vi "bats.parser.test.AddOrderLong.add.oneOrder.vi"(10 "Expected OrderBook.Command[]":T2[](array[typedef])=[{"type"=enum."AddOrder", "side"=66, "orderId "=2319688266934735439, "quantity"=20000, "symbol"=4702127773838221344, "price"=9050, "executed.qty"=0, "canceled.qty"=0, "remaining.qty"=0, "seconds"=0, "nanoseconds"=448000, "Add"=FALSE, "Edit"=FALSE, "Remove"=FALSE}] {"symbol" format="%.0x"; "orderId" format="%.0x"; "side" format="%.0x"}) -> ()   [LabVIEW 2022 SP3]
uses:
  fpga/common/orderbook.command.type.ctl
  fpga/common/orderbook.command.ctl
  pitch/AddOrder/AddOrderLong.Parameters.ctl
  pitch/AddOrder/AddOrderLong.lvclass
panel:
  in  "AddOrderLong.Parameters":T1={"Time Offset"=448000, "Order Id"="ORID001", "Quantity"=20000, "Symbol"="AAPL", "Side Indicator"="B", "Price"=0.905}
  out "Debug":u64[](array[numeric]) format="%.0x"
  out "Passed":bool
  out "OrderBook.Command[]":T2[](array[typedef]) {"remaining.qty" format="%.0x"; "symbol" format="%.0x"; "orderId" format="%.0x"; "side" format="%.0x"}
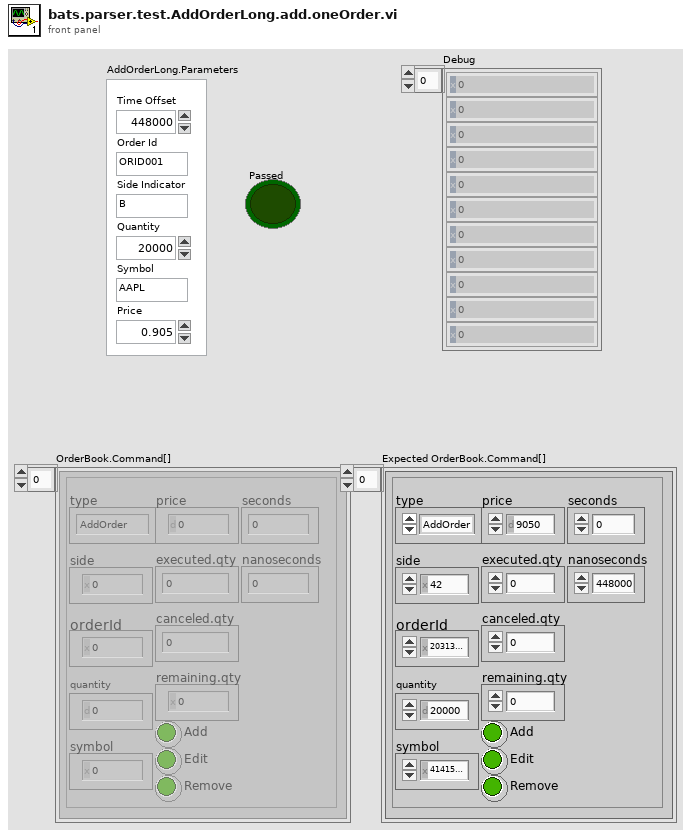
[diagram p1: front panel]
types:
  T1 = typedef "AddOrderLong.lvclass/AddOrderLong.Parameters.ctl" = cluster{"Time Offset":u32, "Order Id":string, "Quantity":u32, "Symbol":string, "Side Indicator":string, "Price":dbl}
  T2 = typedef "orderbook.command.ctl" = cluster{"type":T3, "side":u8, "orderId ":u64, "quantity":u32, "symbol":u64, "price":u64, "executed.qty":u32, "canceled.qty":u32, "remaining.qty":u32, "seconds":u64, "nanoseconds":u64, "Add":bool, "Edit":bool, "Remove":bool}
  T3 = typedef "orderbook.command.type.ctl" = enum8{"Time", "AddOrder", "OrderExecuted", "OrderExecutedAtPrice", "ReduceSize", "ModifyOrder", "DeleteOrder", "Get.Everything", "Get.All.Orders", "Get.Top"}
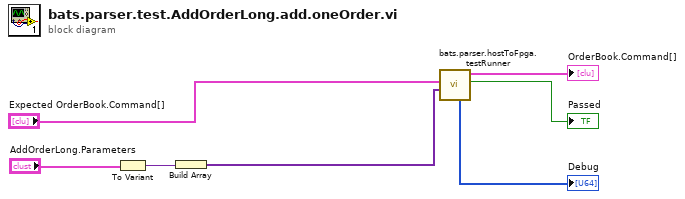
[diagram p0: block diagram]
diagram:
  n1 = To Variant(anything="AddOrderLong.Parameters") -> (Variant=w2:variant)
  n2 = Build Array(w2) -> (w1:variant[])
  n3 = call "bats.parser.hostToFpga.testRunner.vi"("Test.Messages"=w1, "Expected OrderBook.Command[]"="Expected OrderBook.Command[]") -> ("Passed"=→"Passed":bool, "OrderBook.Command[]"=→"OrderBook.Command[]":T2[], "Debug"=→"Debug":u64[])  [unwired: 6 in, 1 out]
